vi "FTW-Endpoint-Connect.vi"(0 "FTW Endpoint":refnum<class "FTW-Endpoint.lvclass">, 5 "Endpoint Address":T1, 11 "error in":errorcluster) -> (4 "FTW Endpoint out":refnum<class "FTW-Endpoint.lvclass">, 15 "error out":errorcluster)   [LabVIEW 2012, in "FTW-Actor.lvlib" / "FTW-Endpoint.lvclass"]
uses:
  FTW-Endpoint.lvclass
  Utility/FTW-Actor-Address.ctl
  FTW-Endpoint.lvclass/FTW-Endpoint.ctl
  FTW-Actor.lvlib
panel:
  # "Inputs"
  # "Outputs"
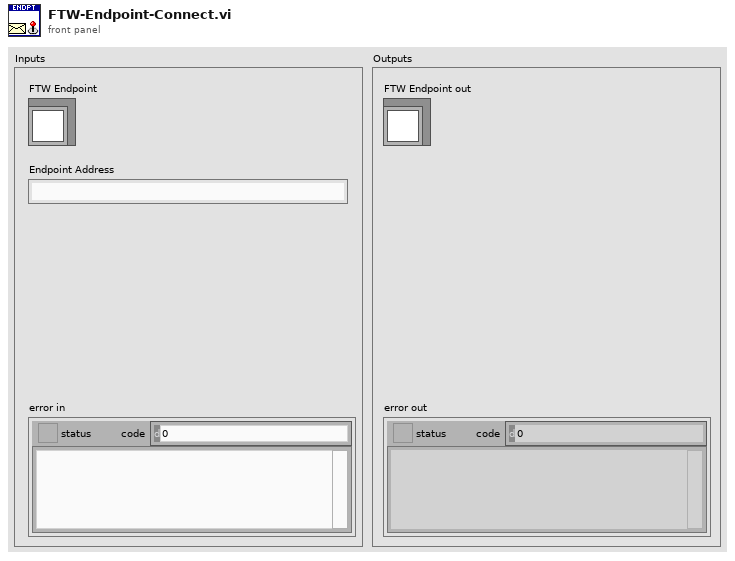
[diagram p1: front panel]
types:
  T1 = typedef "FTW-Actor.lvlib/FTW-Actor-Address.ctl" = string
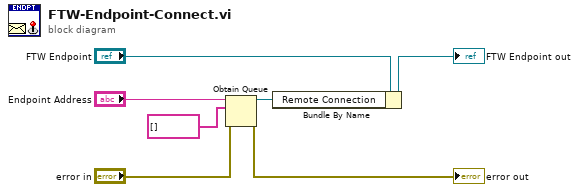
[diagram p0: block diagram]
diagram:
  n1 = Obtain Queue(name (unnamed)="Endpoint Address", element data type=string[] [] ("Multipart Message"), error in (no error)="error in") -> (queue out=w4:refnum<queue>, error out=→"error out":errorcluster)  [unwired: 2 in, 1 out]
  n2 = Bundle By Name(cluster="FTW Endpoint", "Remote Connection"=w4) -> (→"FTW Endpoint out":refnum<class "FTW-Endpoint.lvclass">)
